vi "Update Serial Input.vi"(7 "Serial Input Ref":refnum<vi>, 8 "error in (no error)":errorcluster, 11 "SERIAL INPUT (SI) Ref":refnum<vi>) -> (0 "error out":errorcluster)   [LabVIEW 2025, in "I2C Bus Monitor UI.lvlib"]
uses:
  I2C Bus Monitor UI.lvlib
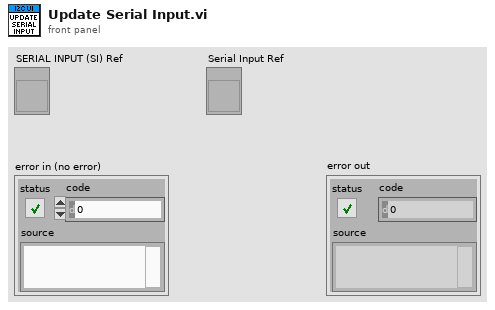
[diagram p1: front panel]
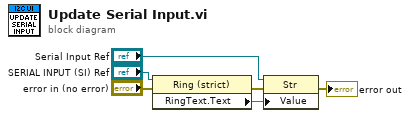
[diagram p0: block diagram]
diagram:
  n1 = property class="Ring (strict)"(reference="SERIAL INPUT (SI) Ref", error in="error in (no error)") -> (error out=w4:errorcluster, "RingText.Text"=w6:string)  [unwired: 1 out]
  n2 = property class="Str"(reference="Serial Input Ref", error in=w4, "Value"=w6) -> (error out=→"error out":errorcluster)  [unwired: 1 out]
